vi "Measure Strain Direct.vi"(7 "ValBufferSize":i32=2048, 8 "error in (no error)":errorcluster {"code" format="%.0x"}, 9 "MaxTime":dbl, 10 "ChannelList":string, 11 "instrument handle":refnum<k15>) -> (0 "error out":errorcluster {"code" format="%.0x"}, 1 "ValActualSize":i32, 2 "Val":dbl[](array[numeric]) format="%.2p", 3 "instrument handle out":refnum<k15>)   [LabVIEW 2020, in "Keysight DAQ970.lvlib"]
doc: "Configures the channels for direct 2-wire strain gauge measurements, immediately sweeps through the specified channels one time (independent of the present scan list), and read the measured data. This command redefines the scan list."
uses:
  Keysight DAQ970.lvlib
  KtDAQ970.dll
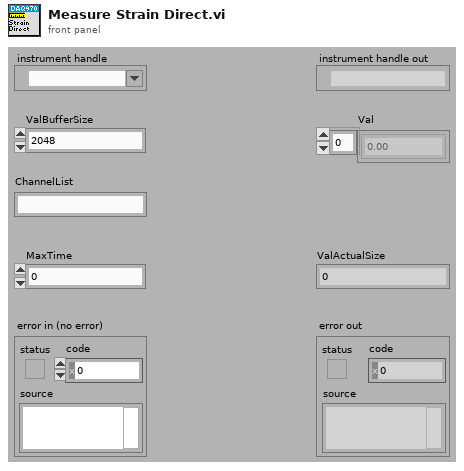
[diagram p1: front panel]
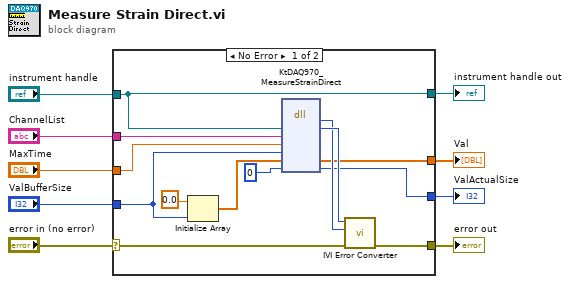
[diagram p0: block diagram]
diagram:
  n1 = case shown="No Error" "error in (no error)" {
    selector: "error in (no error)" -> [w20 w24]
    tunnel: [w19 w24] -> w9
    tunnel: "instrument handle" -> [w10 w23]
    tunnel: "ChannelList" -> [w18 _]
    tunnel: "MaxTime" -> [w17 _]
    tunnel: "ValBufferSize" -> [w11 _]
    tunnel: [w14 _] -> w3
    tunnel: [w12 _] -> w2
    tunnel: [w10 w23] -> w1
    frame No Error {
      n2 = Initialize Array(0.0 ("element"), w11) -> (w16:dbl[])
      n3 = dll-call lib="KtDAQ970**.dll" fn="KtDAQ970_MeasureStrainDirect"("Vi"=w10, "ChannelList"=w18, "MaxTime"=w17, "ValBufferSize"=w11, "Val"=w16, "ValActualSize"=0) -> (w21:i32, "Vi"=w22:u32, "Val"=w14:dbl[], "ValActualSize"=w12:i32)  [unwired: 6 in, 2 out]
      n4 = call "IVI Error Converter.vi"("error in (no error)"=w20, "IVI error code (0)"=w21, "instrument handle"=w22) -> ("error out"=w19:errorcluster)  [unwired: 7 in, 1 out]
    }
    frame Error {
    }
  }
  "error out" <- w9
  "instrument handle out" <- w1
  "Val" <- w3
  "ValActualSize" <- w2
